vi "Write Digital Out.vi"(8 "error in (no error)":errorcluster, 9 "Value":bool, 10 "channel number":u8, 11 "VISA resource name":refnum<visa-resource-name>) -> (0 "error out":errorcluster, 3 "VISA resource name out":refnum<visa-resource-name>)   [LabVIEW 2011, in "Roboteq.lvlib"]
uses:
  Roboteq.lvlib
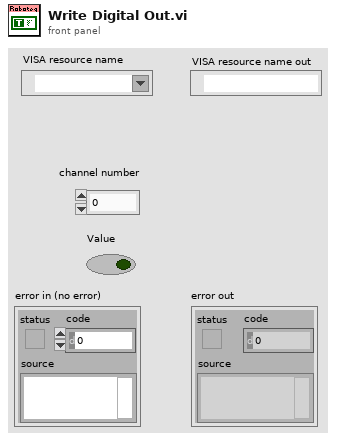
[diagram p1: front panel]
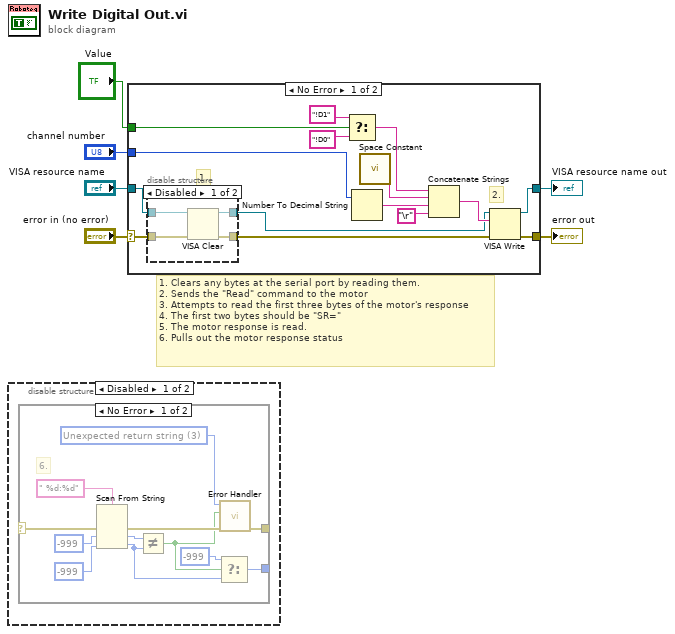
[diagram p0: block diagram]
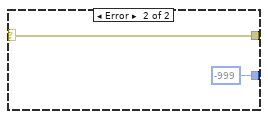
[diagram p2: hidden frame]
diagram:
  # "1. Clears any bytes at the serial port by reading them.\n2. Sends the \"Read\" command to the motor\n3. Attempts to read the first three bytes of the motor's response\n4. The first two bytes should be \"SR=\"\n5. The motor response is read.\n6. Pulls out the motor response status"
  n1 = disable-structure shown="Disabled" {
    frame Disabled {
      n2 = case shown="No Error" {
        selector: _ -> [w16 w19]
        tunnel: [w14 w19] -> _
        tunnel: [w11 -999 ("main battery\nvoltage (V)")] -> _
        frame No Error {
          w12 = u16 3 items=["Scan timeout"=1, "Invalid motor checksum"=2, "Unexpected return string"=3, "Invalid address range"=4] ("Error type")
          # "6."
          n3 = Scan From String(format string=" %d:%d", error in=w16, default 1=-999 ("default value 1"), default 2=-999 ("default value 1")) -> (error out=w13:errorcluster, output 1=w10:i32, output 2=w7:i32)  [unwired: 2 in, 2 out]
          n4 = Not Equal?(x=w10, y=w7) -> (x != y?=w8:bool)
          n5 = Select(t=-999 ("default value 1"), s=w8, f=w7) -> (s? t:f=w11:i32)
          n6 = call "Error Handler.vi"("error in (no error)"=w13, "Error? (no error)"=w8, "Error type"=w12) -> ("error out"=w14:errorcluster)  [unwired: 8 in]
        }
        frame Error {
        }
      }
    }
    frame Enabled {
    }
  }
  n7 = case shown="No Error" "error in (no error)" {
    selector: "error in (no error)" -> [w31 w43]
    tunnel: [w21 w43] -> w5
    tunnel: "VISA resource name" -> [w32 w42]
    tunnel: [w22 w42] -> w3
    tunnel: "channel number" -> [w33 _]
    tunnel: "Value" -> [w28 _]
    frame No Error {
      # "2."
      # "1."
      n8 = disable-structure shown="Disabled" {
        disable-tunnel: w32 -> [w39 w40]
        disable-tunnel: w31 -> [w38 w41]
        disable-tunnel: [w37 w40] -> w30
        disable-tunnel: [w36 w41] -> w29
        frame Disabled {
          n9 = VISA Clear(VISA resource name=w39, error in (no error)=w38) -> (VISA resource name out=w37:refnum<visa-resource-name>, error out=w36:errorcluster)
        }
        frame Enabled {
        }
      }
      n10 = Select(t="!D1" ("string"), s=w28, f="!D0" ("string")) -> (s? t:f=w23:string)
      n11 = Number To Decimal String(number=w33) -> (decimal integer string=w27:string)  [unwired: 1 in]
      n12 = call <vilib>:"Space Constant.vi"() -> ("String"=w26:string)
      n13 = Concatenate Strings(w23, w26, w27, "\r") -> (w35:string)
      n14 = VISA Write(VISA resource name=w30, write buffer=w35, error in (no error)=w29) -> (VISA resource name out=w22:refnum<visa-resource-name>, error out=w21:errorcluster)  [unwired: 1 out]
    }
    frame Error {
    }
  }
  "VISA resource name out" <- w3
  "error out" <- w5
